vi "Static noise.vi"(1 "Fraction":dbl, 2 "Input":dbl) -> (0 "Output with noise":dbl)   [LabVIEW 2018]
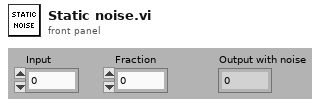
[diagram p1: front panel]
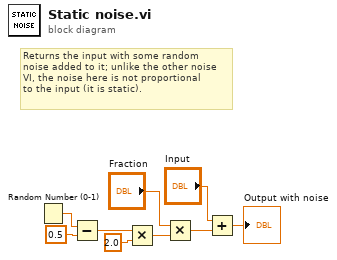
[diagram p0: block diagram]
diagram:
  # "Returns the input with some random\nnoise added to it; unlike the other noise\nVI, the noise here is not proportional\nto the input (it is static)."
  n1 = Random Number (0-1)() -> (number: 0 to 1=w6:dbl)
  n2 = Subtract(x=w6, y=0.5) -> (x-y=w4:dbl)
  n3 = Multiply(x=w4, y=2.0) -> (x*y=w2:dbl)
  n4 = Multiply(x="Fraction", y=w2) -> (x*y=w7:dbl)
  n5 = Add(x="Input", y=w7) -> (x+y=→"Output with noise":dbl)
